vi "PSTR-Initialize.vi"(0 "PSTR Params":T2={"Stimulus"={"Ear"=enum."Right", "BW (oct)"=0.0, "Seed"=0, "Ramp (ms)"=0.0, "On time (ms)"=0.0, "Off time (ms)"=0.0, "Delay (ms)"=10000.0}, "FreqSeq"={"Min (kHz)"=0.0, "Max (kHz)"=0.0, "Step (oct)"=0.0}, "LevelSeq"={"Min (dB)"=0.0, "Max (dB)"=0.0, "Step (dB)"=0.0}, "Seq"={"Order"=enum."Sequential", "Averages"=0}, "Response"={"Grass gain"=0.0, "Window (ms)"=0.0}, "Hidden"={"Sample rate (Hz)"=0.0, "Nfft"=0, "save raw"=FALSE, "sep"=0.0, "Window"=enum."NONE"}, "RejThr"=0.0}, 1 "Data folder":path, 7 "Freq (kHz)":dbl, 11 "error in (no error)":errorcluster) -> (4 "Runtime":T1 {"window" items=["None ", "Hanning", "Hamming", "Blackman-Harris", "Exact Blackman", "Blackman", "Flat Top", "4 Term B-Harris ", "7 Term B-Harris", "Low Sidelobe"]}, 15 "error out":errorcluster)   [LabVIEW 2020]
uses:
  Typedefs/PSTR-Parameters.ctl
  Typedefs/PSTR-Stimulus Params.ctl
  Typedefs/PSTR-FreqSeq Params.ctl
  Typedefs/PSTR-LevelSeq Params.ctl
  Typedefs/PSTR-SeqParams.ctl
  Typedefs/PSTR-Response Params.ctl
  Typedefs/PSTR-Hidden Params.ctl
  Typedefs/PSTR-Window Shape.ctl
  Typedefs/PSTR-Runtime Data.ctl
  epl-vi-lib/Signal Synthesis VIs/4th Generation/Classes/SignalManager/SignalManager.lvclass
  epl-vi-lib/Signal Synthesis VIs/4th Generation/Classes/Filter/Shape.ctl
  epl-vi-lib/Signal Synthesis VIs/4th Generation/Classes/Filter/Units.ctl
  epl-vi-lib/Signal Synthesis VIs/4th Generation/Classes/Filter/Class.ctl
  epl-vi-lib/Signal Synthesis VIs/4th Generation/Classes/Level/LevelUnits.ctl
  epl-vi-lib/Signal Synthesis VIs/4th Generation/Classes/Gate/Shape.ctl
  epl-vi-lib/Signal Synthesis VIs/4th Generation/Classes/Gate/Gate.lvclass/Gate.ctl
  epl-vi-lib/Signal Synthesis VIs/4th Generation/Classes/Filter/Filter.lvclass/Filter.ctl
  epl-vi-lib/Signal Synthesis VIs/4th Generation/Classes/Waveforms/Noise/Noise.lvclass/Noise.ctl
  epl-vi-lib/Signal Synthesis VIs/4th Generation/Classes/Channel/Channel.lvclass/Channel.ctl
  c8a47efb-eddf-4299-852e-93ddb79bc2f1.vi
  0b68258d-870d-4f2d-a2e2-9ff453b5e453.vi
  de9fc71a-c8e6-4afe-ad44-ab5690ffd704.vi
  4f0ed9b9-7547-4d7f-91c8-e8713f57b3e7.vi
  44352459-fa99-4d29-a9e0-a1d4e78b3677.vi
  epl-vi-lib/Signal Synthesis VIs/4th Generation/Classes/Gate/Write Shape.vi
  epl-vi-lib/Signal Synthesis VIs/4th Generation/Classes/Filter/Write Type.vi
  epl-vi-lib/Signal Synthesis VIs/4th Generation/Classes/Filter/Write Units.vi
  epl-vi-lib/Signal Synthesis VIs/4th Generation/Classes/Filter/Write BW (kHz).vi
  epl-vi-lib/Signal Synthesis VIs/4th Generation/Classes/Filter/Write Cascade.vi
  epl-vi-lib/Signal Synthesis VIs/4th Generation/Classes/Filter/Write Class.vi
  epl-vi-lib/Signal Synthesis VIs/4th Generation/Classes/Filter/Write Order.vi
  epl-vi-lib/Signal Synthesis VIs/4th Generation/Classes/Filter/Write CF (kHz).vi
  epl-vi-lib/Signal Synthesis VIs/4th Generation/Classes/Waveforms/Noise/Write Seed.vi
  epl-vi-lib/Signal Synthesis VIs/4th Generation/Classes/Channel/Write Waveform.vi
  epl-vi-lib/Signal Synthesis VIs/4th Generation/Classes/Channel/Write Filter.vi
  epl-vi-lib/Signal Synthesis VIs/4th Generation/Classes/Channel/Write Gate.vi
  epl-vi-lib/Signal Synthesis VIs/4th Generation/Classes/Channel/Write Level.vi
  epl-vi-lib/Signal Synthesis VIs/4th Generation/Classes/Channel/Write AltPol.vi
  epl-vi-lib/Signal Synthesis VIs/4th Generation/Classes/Waveforms/Noise/Noise.lvclass
  D:/Development/epl-vi-lib/Signal Synthesis VIs/4th Generation/Classes/Waveforms/Waveform/Waveform.lvclass
  epl-vi-lib/Utility VIs/Math VIs/LinSpace (start-stop-step).vi
  <vilib>/Utility/config.llb/Open Config Data.vi
  <vilib>/Utility/config.llb/Get Key Names.vi
  <vilib>/Utility/config.llb/Read Key.vi
  <vilib>/Utility/config.llb/Read Key (String).vi
  epl-vi-lib/Utility VIs/Array Manipulation VIs/String Array to Comma Separated String.vi
  <vilib>/Utility/error.llb/Error Cluster From Error Code.vi
  <vilib>/Utility/config.llb/Close Config Data.vi
  epl-vi-lib/PXI DAQ VIs/AODO/AODO-Engine.vi
  epl-vi-lib/PXI DAQ VIs/AIDI/AIDI-Engine.vi
  epl-vi-lib/Utility VIs/Array Manipulation VIs/Irregular Array Subset (DBL).vi
  epl-vi-lib/Signal Synthesis VIs/4th Generation/Classes/Gate/Gate.lvclass
  epl-vi-lib/Signal Synthesis VIs/4th Generation/Classes/Channel/Channel.lvclass
  epl-vi-lib/Signal Synthesis VIs/4th Generation/Classes/Filter/Filter.lvclass
  epl-vi-lib/Signal Synthesis VIs/4th Generation/Classes/Level/Level.lvclass
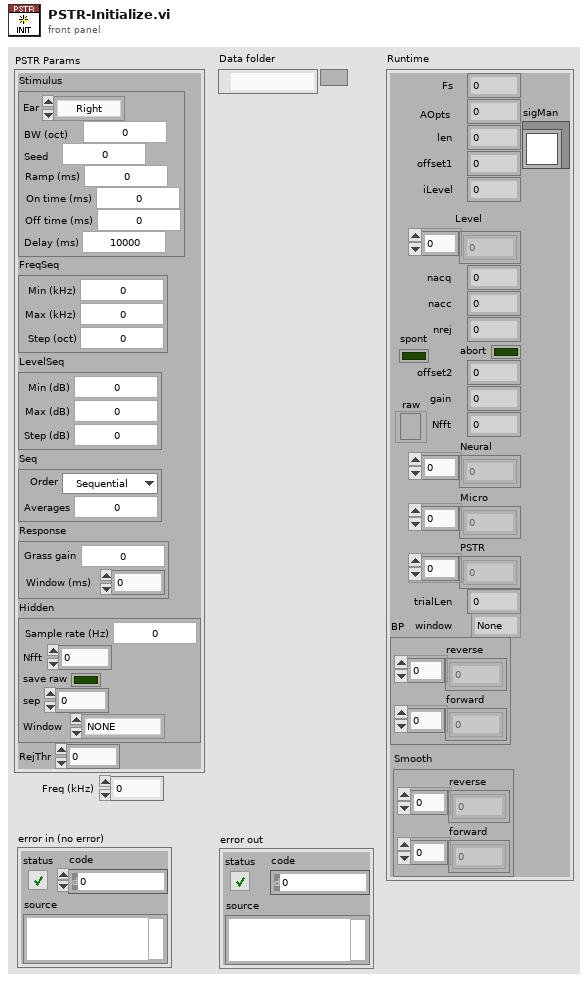
[diagram p1: front panel]
types:
  T1 = typedef "PSTR-Runtime Data.ctl" = cluster{"Fs":dbl, "AOpts":i32, "len":i32, "offset1":i32, "iLevel":i32, "Level":dbl[], "nacc":i32, "nrej":i32, "nacq":i32, "abort":bool, "offset2":i32, "gain":dbl, "Nfft":i32, "Neural":dbl[], "Micro":dbl[], "raw":refnum<file>, "spont":bool, "PSTR":dbl[], "trialLen":i32, "window":u16, "BP":cluster{"reverse":dbl[], "forward":dbl[]}, "Smooth":cluster{"reverse":dbl[], "forward":dbl[]}, "sigMan":refnum<class "SignalManager.lvclass">}
  T2 = typedef "PSTR-Parameters.ctl" = cluster{"Stimulus":T3, "FreqSeq":T4, "LevelSeq":T5, "Seq":T6, "Response":T7, "Hidden":T8, "RejThr":dbl}
  T3 = typedef "PSTR-Stimulus Params.ctl" = cluster{"Ear":enum16{"Right", "Left"}, "BW (oct)":dbl, "Seed":i32, "Ramp (ms)":dbl, "On time (ms)":dbl, "Off time (ms)":dbl, "Delay (ms)":dbl}
  T4 = typedef "PSTR-FreqSeq Params.ctl" = cluster{"Min (kHz)":dbl, "Max (kHz)":dbl, "Step (oct)":dbl}
  T5 = typedef "PSTR-LevelSeq Params.ctl" = cluster{"Min (dB)":dbl, "Max (dB)":dbl, "Step (dB)":dbl}
  T6 = typedef "PSTR-SeqParams.ctl" = cluster{"Order":enum16{"Sequential", "Random"}, "Averages":i32}
  T7 = typedef "PSTR-Response Params.ctl" = cluster{"Grass gain":dbl, "Window (ms)":dbl}
  T8 = typedef "PSTR-Hidden Params.ctl" = cluster{"Sample rate (Hz)":dbl, "Nfft":i32, "save raw":bool, "sep":dbl, "Window":T9}
  T9 = typedef "PSTR-Window Shape.ctl" = enum16{"NONE", "Hamming"}
  T10 = typedef "Gate.lvclass/Shape.ctl" = enum16{"OFF", "Rectangle", "Sine-squared", "Trapezoid"}
  T11 = typedef "Level.lvclass/LevelUnits.ctl" = enum16{"dB atten", "dB SPL", "dB Vrms", "Volts", "dB mW", "mW", "dB HL", "dB SL"}
  T12 = typedef "Filter.lvclass/Class.ctl" = enum16{"Elliptic", "Butterworth", "Brickwall"}
  T13 = typedef "Filter.lvclass/Units.ctl" = enum16{"Linear", "Octaves", "Min-Max"}
  T14 = typedef "Filter.lvclass/Shape.ctl" = enum16{"OFF", "Lowpass", "Highpass", "Bandpass", "Bandstop"}
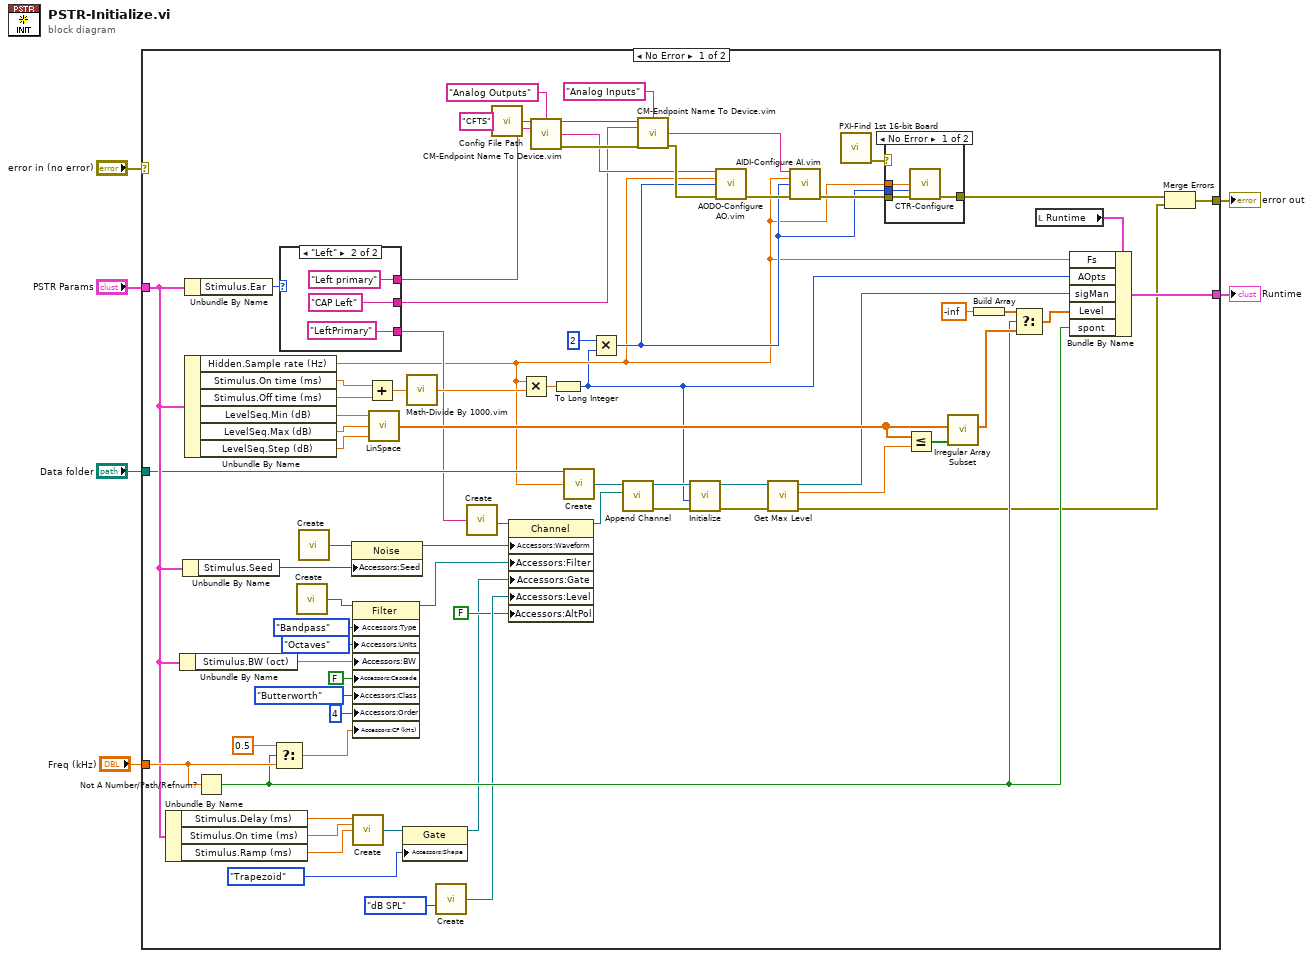
[diagram p0: block diagram]
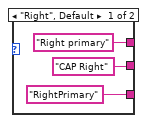
[diagram p3: hidden frame]
diagram:
  n1 = case shown="No Error" "error in (no error)" {
    selector: "error in (no error)" -> [_ w92]
    tunnel: "PSTR Params" -> [w58 _]
    tunnel: [w66 w92] -> w6
    tunnel: [w73 _] -> w3
    tunnel: "Freq (kHz)" -> [w65 _]
    tunnel: "Data folder" -> [w39 _]
    frame No Error {
      n2 = Unbundle By Name(w58) -> ("Stimulus.Delay (ms)"=w44:dbl, "Stimulus.On time (ms)"=w34:dbl, "Stimulus.Ramp (ms)"=w33:dbl)
      n3 = Unbundle By Name(w58) -> ("Stimulus.BW (oct)"=w50:dbl)
      n4 = Unbundle By Name(w58) -> ("Stimulus.Seed"=w55:i32)
      n5 = Unbundle By Name(w58) -> ("Stimulus.Ear"=w80:enum16{"Right", "Left"})
      n6 = Unbundle By Name(w58) -> ("Hidden.Sample rate (Hz)"=w15:dbl, "Stimulus.On time (ms)"=w79:dbl, "Stimulus.Off time (ms)"=w78:dbl, "LevelSeq.Min (dB)"=w71:dbl, "LevelSeq.Max (dB)"=w70:dbl, "LevelSeq.Step (dB)"=w69:dbl)
      n7 = Not A Number/Path/Refnum?(number/path/refnum=w65) -> (NaN/Path/Refnum?=w59:bool)
      n8 = Select(t=0.5, s=w59, f=w65) -> (s? t:f=w45:dbl)
      n9 = case shown="\"Left\"" w80 {
        tunnel: ["RightPrimary" "LeftPrimary"] -> w20
        tunnel: ["Right primary" "Left primary"] -> w19
        tunnel: ["CAP Right" "CAP Left"] -> w18
        frame "Right", Default {
        }
        frame "Left" {
        }
      }
      n10 = call "Create.vi"() -> ("Filter"=w53:refnum<class "Filter.lvclass">)  [unwired: 15 in]
      n11 = call "Create.vi"() -> ("Noise"=w56:refnum<class "Noise.lvclass">)  [unwired: 15 in]
      n12 = property class="Noise"(reference=w56, "Accessors:Seed"=w55) -> (reference out=w54:refnum<class "Noise.lvclass">)  [unwired: 1 in, 1 out]
      n13 = property class="Filter"(reference=w53, "Accessors:Type"=Shape."Bandpass" ("Type"), "Accessors:Units"=Units."Octaves" ("Units"), "Accessors:BW"=w50, "Accessors:Cascade"=FALSE ("Cascade"), "Accessors:Class"=Class."Butterworth" ("Class"), "Accessors:Order"=4 ("Order"), "Accessors:CF (kHz)"=w45) -> (reference out=w49:refnum<class "Filter.lvclass">)  [unwired: 1 in, 1 out]
      n14 = call "Create.vi"("Delay (ms)"=w44, "Duration (ms)"=w34, "Ramp (ms)"=w33) -> ("Gate"=w43:refnum<class "Gate.lvclass">)  [unwired: 12 in]
      n15 = Add(x=w79, y=w78) -> (x+y=w77:dbl)
      n16 = call-poly "LinSpace.vi"("Step"=w69, "Stop"=w70, "Start"=w71) -> ("Array"=w67:dbl[])  [unwired: 1 in, 1 out]
      n17 = property class="Gate"(reference=w43, "Accessors:Shape"=Shape."Trapezoid" ("Shape")) -> (reference out=w36:refnum<class "Gate.lvclass">)  [unwired: 1 in, 1 out]
      n18 = call "Math-Divide By 1000.vim"("X"=w77) -> ("1000X"=w76:dbl)
      n19 = call "Create.vi"("Units"=LevelUnits."dB SPL") -> ("Level"=w41:refnum<class "Level.lvclass">)  [unwired: 14 in]
      n20 = call "Create.vi"("Name"=w20) -> ("Channel"=w57:refnum<class "Channel.lvclass">)  [unwired: 14 in]
      n21 = call "Config File Path.vi"("AppName"="CFTS") -> ("Default config file name"=w21:path)
      n22 = property class="Channel"(reference=w57, "Accessors:Waveform"=w54, "Accessors:Filter"=w49, "Accessors:Gate"=w36, "Accessors:Level"=w41, "Accessors:AltPol"=FALSE ("AltPol")) -> (reference out=w37:refnum<class "Channel.lvclass">)  [unwired: 1 in, 1 out]
      n23 = Multiply(x=w15, y=w76) -> (x*y=w75:dbl)
      n24 = call "CM-Endpoint Name To Device.vim"("Path"=w21, "IO Type"="Analog Outputs", "Names in"=w19) -> ("Path thru"=w29:path, "Devices"=w26:string, "error out"=w28:errorcluster)  [unwired: 9 in, 1 out]
      n25 = To Long Integer(number=w75) -> (32bit integer=w12:i32)
      n26 = call "Create.vi"("Cal Folder"=w39, "Fs (Hz)"=w15) -> ("SigMan"=w38:refnum<class "SignalManager.lvclass">)  [unwired: 13 in]
      n27 = Multiply(x=2, y=w12) -> (x*y=w17:i32)
      n28 = call "Append Channel.vi"("Channel"=w37, "SignalManager in"=w38) -> ("error out"=w13:errorcluster, "SignalManager out"=w14:refnum<class "SignalManager.lvclass">)  [unwired: 8 in]
      n29 = call "CM-Endpoint Name To Device.vim"("Path"=w29, "IO Type"="Analog Inputs", "Names in"=w18, "error in (no error)"=w28) -> ("Devices"=w24:string, "error out"=w27:errorcluster)  [unwired: 8 in, 2 out]
      n30 = call "Initialize.vi"("error in (no error)"=w13, "Npts"=w12, "SigMan in"=w14) -> ("error out"=w10:errorcluster, "SigMan out"=w11:refnum<class "SignalManager.lvclass">)  [unwired: 7 in]
      n31 = call "AODO-Configure AO.vim"("AO.Channels"=w26, "AO.Fs (Hz)"=w15, "AO.Npts"=w17, "error in (no error)"=w27) -> ("error out"=w25:errorcluster)  [unwired: 11 in]
      n32 = call "Get Max Level.vi"("error in (no error)"=w10, "SignalManager in"=w11) -> ("error out"=w9:errorcluster, "Max level"=w7:dbl, "SignalManager out"=w8:refnum<class "SignalManager.lvclass">)  [unwired: 7 in]
      n33 = call "AIDI-Configure AI.vim"("AI.Channels"=w24, "AI.Fs (Hz)"=w15, "AI.Npts"=w17, "error in (no error)"=w25) -> ("error out"=w23:errorcluster)  [unwired: 11 in]
      n34 = call "PXI-Find 1st 16-bit Board.vi"() -> ("error out"=w22:errorcluster)  [unwired: 9 in, 2 out]
      n35 = case shown="No Error" w22 {
        tunnel: w23 -> [w84 w85]
        tunnel: w15 -> [w83 _]
        tunnel: w17 -> [w82 _]
        tunnel: [w81 w85] -> w16
        frame No Error {
          n36 = call "CTR-Configure.vi"("Sampling rate (Hz)"=w83, "Npts"=w82, "error in (no error)"=w84) -> ("error out"=w81:errorcluster)  [unwired: 12 in]
        }
        frame Error {
        }
      }
      n37 = Less Or Equal?(x=w67, y=w7) -> (x <= y?=w68:bool[])
      n38 = call-poly "Irregular Array Subset.vi"("Mask"=w68, "Array"=w67) -> ("Array Subset"=w61:dbl[])  [unwired: 8 in, 1 out]
      n39 = Build Array(-inf) -> (w62:dbl[])
      n40 = Select(t=w62, s=w59, f=w61) -> (s? t:f=w60:dbl[])
      n41 = local read "Runtime"() -> (w74:T1)
      n42 = Bundle By Name(cluster=w74, "Fs"=w15, "AOpts"=w12, "sigMan"=w8, "Level"=w60, "spont"=w59) -> (w73:T1)
      n43 = Merge Errors(w16, w9) -> (w66:errorcluster)
    }
    frame Error {
    }
  }
  "error out" <- w6
  "Runtime" <- w3
